vi "display_tree.vi"(8 "error in (no error)":errorcluster, 9 "parent tag":string, 10 "XML tree":refnum<vi>, 11 "Element in":refnum<class "XMLElement.lvclass">=refnum) -> (0 "error out":errorcluster, 3 "Element out":refnum<class "XMLElement.lvclass">)   [LabVIEW 2010]
uses:
  bricks/classes/XMLElement/XMLElement/XMLElement.lvclass
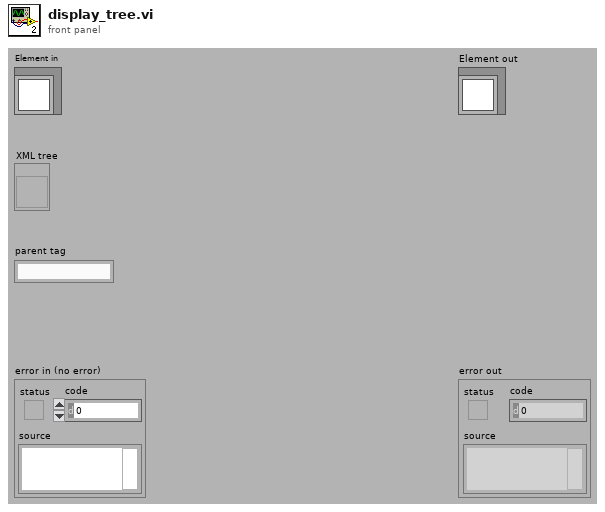
[diagram p1: front panel]
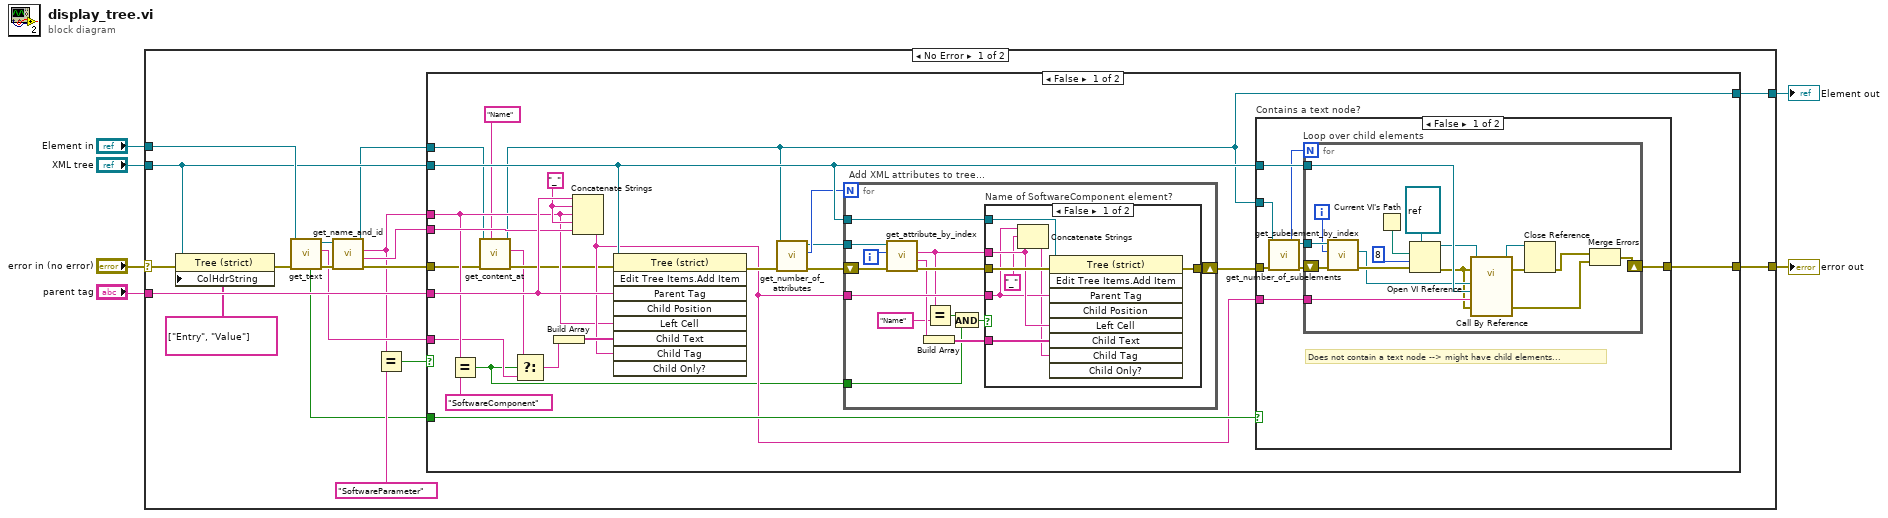
[diagram p0: block diagram]
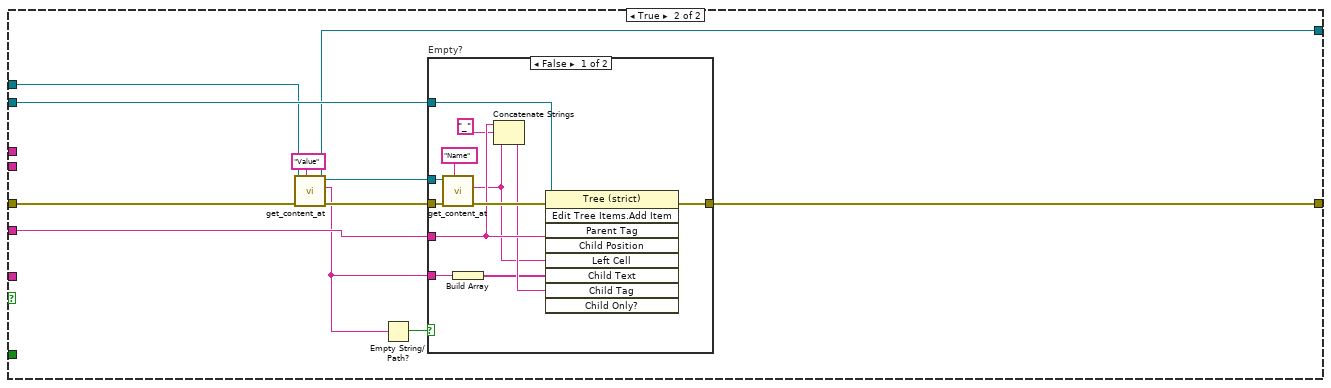
[diagram p4: hidden frame]
diagram:
  n1 = case shown="No Error" "error in (no error)" {
    selector: "error in (no error)" -> [w22 w122]
    tunnel: [w24 w122] -> w5
    tunnel: [w8 w121] -> w3
    tunnel: "Element in" -> [w19 w121]
    tunnel: "XML tree" -> [w11 _]
    tunnel: "parent tag" -> [w21 _]
    frame No Error {
      n2 = property class="Tree (strict)"(reference=w11, error in=w22, "ColHdrString"=string[] ["Entry", "Value"] ("Column Header Strings[]")) -> (error out=w15:errorcluster)  [unwired: 1 out]
      n3 = call "get_text.vi"("error in (no error)"=w15, "Element in"=w19) -> ("error out"=w20:errorcluster, "text"=w16:string, "Element out"=w18:refnum<class "XMLElement.lvclass">, "text node?"=w10:bool)  [unwired: 6 in]
      n4 = call "get_name_and_id.vi"("error in (no error)"=w20, "Element in"=w18) -> ("error out"=w23:errorcluster, "ID"=w17:string, "name"=w12:string, "Element out"=w7:refnum<class "XMLElement.lvclass">)  [unwired: 6 in]
      n5 = Equal?(x=w12, y="SoftwareParameter" ("x")) -> (x = y?=w9:bool)
      n6 = case shown="False" w9 {
        tunnel: [w48 w107] -> w24
        tunnel: w23 -> [w31 w99]
        tunnel: w21 -> [w47 w105]
        tunnel: w17 -> [w46 _]
        tunnel: w16 -> [w27 _]
        tunnel: w12 -> [w34 _]
        tunnel: w11 -> [w44 w106]
        tunnel: w10 -> [w43 _]
        tunnel: w7 -> [w33 w100]
        tunnel: [w32 w101] -> w8
        frame False {
          w37 = "_"
          n7 = Equal?(x=w34, y="SoftwareComponent" ("x")) -> (x = y?=w25:bool)
          n8 = call "get_content_at.vi"("attribute name"="Name", "error in (no error)"=w31, "Element in"=w33) -> ("error out"=w30:errorcluster, "string"=w28:string, "Element out"=w32:refnum<class "XMLElement.lvclass">)  [unwired: 5 in, 1 out]
          n9 = Select(t=w28, s=w25, f=w27) -> (s? t:f=w26:string)
          n10 = Build Array(w26) -> (w41:string[])
          n11 = Concatenate Strings(w47, w37, w34, w37, w46) -> (w36:string)
          n12 = invoke class="Tree (strict)" method="Edit Tree Items.Add Item"(reference=w44, error in=w30, "Parent Tag"=w47, "Left Cell"=w34, "Child Text"=w41, "Child Tag"=w36) -> (error out=w42:errorcluster)  [unwired: 3 in, 8 out]
          n13 = call "get_number_of_attributes.vi"("error in (no error)"=w42, "XMLElement in"=w32) -> ("error out"=w40:errorcluster, "number of attributes"=w39:i32, "XMLElement out"=w38:refnum<class "XMLElement.lvclass">)  [unwired: 6 in, 1 out]
          n14 = for "Add XML attributes to tree..." {
            N: w39 -> [_]
            shift-right: [w58] -> w45
            shift-left: w40 -> [w62]
            tunnel: w38 -> [w60]
            tunnel: w44 -> [w57]
            tunnel: w36 -> [w56]
            tunnel: w25 -> [w51]
            i -> [w61]
            n15 = call "get_attribute_by_index.vi"("error in (no error)"=w62, "index"=w61, "XMLElement in"=w60) -> ("error out"=w59:errorcluster, "value"=w54:string, "name"=w49:string)  [unwired: 5 in, 1 out]
            n16 = Build Array(w54) -> (w55:string[])
            n17 = Equal?(x=w49, y="Name") -> (x = y?=w52:bool)
            n18 = And(x=w52, y=w51) -> (x .and. y?=w50:bool)
            n19 = case "Name of SoftwareComponent element?" shown="False" w50 {
              tunnel: w59 -> [w70 w71]
              tunnel: [w69 w71] -> w58
              tunnel: w57 -> [w68 _]
              tunnel: w49 -> [w67 _]
              tunnel: w56 -> [w66 _]
              tunnel: w55 -> [w65 _]
              frame False {
                n20 = Concatenate Strings(w66, "_", w67) -> (w63:string)
                n21 = invoke on="Invoke Node" class="Tree (strict)" method="Edit Tree Items.Add Item"(reference=w68, error in=w70, "Parent Tag"=w66, "Left Cell"=w67, "Child Text"=w65, "Child Tag"=w63) -> (error out=w69:errorcluster)  [unwired: 3 in, 8 out]
              }
              frame True {
                # "Don't display..."
              }
            }
          }
          n22 = case "Contains a text node?" shown="False" w43 {
            tunnel: [w79 w97] -> w48
            tunnel: w44 -> [w78 _]
            tunnel: w36 -> [w77 _]
            tunnel: w45 -> [w76 w97]
            tunnel: w32 -> [w73 _]
            frame False {
              # "Does not contain a text node --> might have child elements..."
              n23 = call "get_number_of_subelements.vi"("error in (no error)"=w76, "Element in"=w73) -> ("error out"=w75:errorcluster, "number of subelements"=w72:i32, "Element out"=w74:refnum<class "XMLElement.lvclass">)  [unwired: 6 in, 1 out]
              n24 = for "Loop over child elements" {
                N: w72 -> [_]
                shift-right: [w92] -> w79
                shift-left: w75 -> [w96]
                tunnel: w74 -> [w95]
                tunnel: w78 -> [w93]
                tunnel: w77 -> [w91]
                i -> [w94]
                n25 = call "get_subelement_by_index.vi"("error in (no error)"=w96, "index"=w94, "Element in"=w95) -> ("error out"=w90:errorcluster, "subelement"=w89:refnum<class "XMLElement.lvclass">)  [unwired: 5 in, 2 out]
                n26 = Current VI's Path() -> (path=w83:path)
                n27 = Open VI Reference(type specifier VI Refnum (for type only)=refnum<vi> refnum, vi path=w83, options=8, error in (no error)=w90) -> (vi reference=w87:refnum<vi>, error out=w85:errorcluster)  [unwired: 2 in]
                n28 = call-by-ref "?"(reference=w87, error in=w85, 8:"error in (no error)"=w85, "parent tag"=w91, "XML tree"=w93, "Element in"=w89) -> (reference out=w80:refnum<vi>, error out=w82:errorcluster, 0:"error out"=w88:errorcluster)  [unwired: 6 in, 1 out]
                n29 = Close Reference(reference=w80, error in (no error)=w82) -> (error out=w81:errorcluster)
                n30 = Merge Errors(w81, w88) -> (w92:errorcluster)
              }
            }
            frame True {
            }
          }
        }
        frame True {
          n31 = call "get_content_at.vi"("attribute name"="Value", "error in (no error)"=w99, "Element in"=w100) -> ("error out"=w103:errorcluster, "string"=w98:string, "Element out"=w101:refnum<class "XMLElement.lvclass">)  [unwired: 5 in, 1 out]
          n32 = Empty String/Path?(string/path=w98) -> (empty?=w102:bool)
          n33 = case "Empty?" shown="False" w102 {
            tunnel: [w119 w120] -> w107
            tunnel: w106 -> [w118 _]
            tunnel: w105 -> [w113 _]
            tunnel: w103 -> [w117 w120]
            tunnel: w98 -> [w109 _]
            tunnel: w101 -> [w114 _]
            frame False {
              n34 = call "get_content_at.vi"("attribute name"="Name", "error in (no error)"=w117, "Element in"=w114) -> ("error out"=w116:errorcluster, "string"=w110:string)  [unwired: 5 in, 2 out]
              n35 = Build Array(w109) -> (w108:string[])
              n36 = Concatenate Strings(w113, "_", w110) -> (w111:string)
              n37 = invoke on="Invoke Node" class="Tree (strict)" method="Edit Tree Items.Add Item"(reference=w118, error in=w116, "Parent Tag"=w113, "Left Cell"=w110, "Child Text"=w108, "Child Tag"=w111) -> (error out=w119:errorcluster)  [unwired: 3 in, 8 out]
            }
            frame True {
            }
          }
        }
      }
    }
    frame Error {
    }
  }
  "error out" <- w5
  "Element out" <- w3
